vi "Read.vi"(8 "error in (no error)":errorcluster, 11 "Numeric in":refnum<class "Const_I8.lvclass">) -> (0 "error out":errorcluster, 2 "Numeric":T1, 3 "Numeric out":refnum<class "Const_I8.lvclass">)   [LabVIEW 2021, in "Const_I8.lvclass"]
uses:
  Const_I8.lvclass
  Type.ctl
  Const_I8.lvclass/Const_I8.ctl
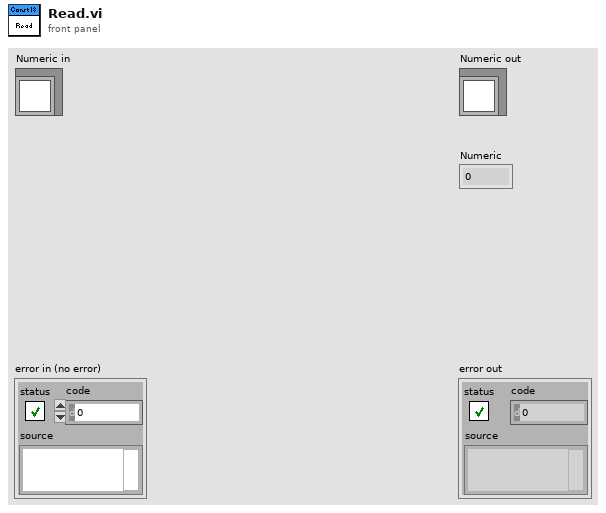
[diagram p1: front panel]
types:
  T1 = typedef "Const_I8.lvclass/Type.ctl" = i8
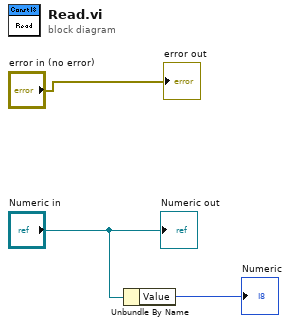
[diagram p0: block diagram]
diagram:
  n1 = Unbundle By Name("Numeric in") -> ("Value"=→"Numeric":T1)
  "error out" <- "error in (no error)"
  "Numeric out" <- "Numeric in"
